vi "Client.vi"   [LabVIEW 2013]
uses:
  <vilib>/NXT/Block Support/NXT_MessageMailbox.ctl
  <vilib>/NXT/Dual Mode Library/Display/drawText.vi
  <vilib>/NXT/Dual Mode Library/BT/BlueTooth_Write_String.vi
types:
  T1 = typedef "LVHSConnector.ctl" = refnum<class "BrickReference.lvclass">
  T2 = typedef "NXT_MessageMailbox.ctl" = u8
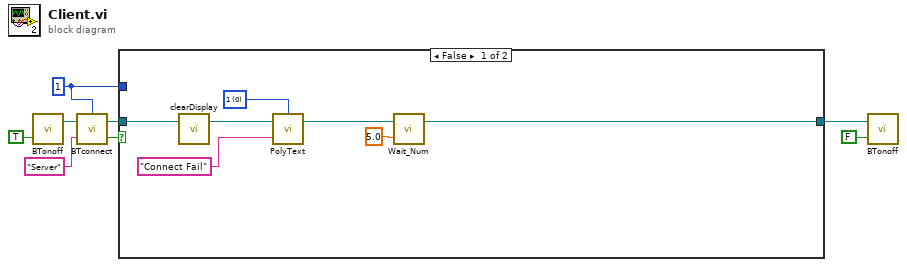
[diagram p0: block diagram]
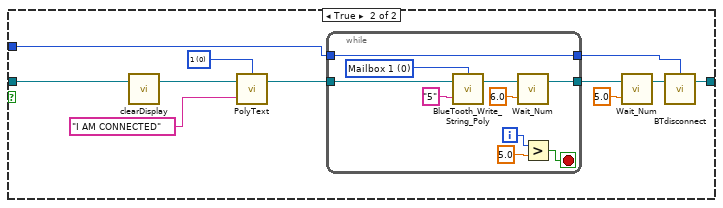
[diagram p2: hidden frame]
diagram:
  w5 = u8 1 ("Connection")
  n1 = call <vilib>:"BTonoff.vi"("On/Off"=TRUE) -> ("NXT/EV3"=w8:T1)  [unwired: 2 in, 1 out]
  n2 = call <vilib>:"BTconnect.vi"("Partner Name"="Server", "NXT/EV3"=w8, "Connection"=w5) -> ("Success"=w2:bool, "NXT/EV3"=w3:T1)
  n3 = case shown="False" w2 {
    tunnel: w5 -> [_ w19]
    tunnel: [w9 w26] -> w4
    tunnel: w3 -> [w10 w20]
    frame False {
      w13 = i16 0 items=["1", "2", "3", "4", "5", "6", "7", "8", "9", "10", "11", "12"] ("Line")
      n4 = call <vilib>:"clearDisplay.vi"("NXT/EV3"=w10) -> ("NXT/EV3"=w15:T1)  [unwired: 3 in]
      n5 = call-poly <vilib>:"PolyText.vi"("Text"="Connect Fail", "NXT/EV3"=w15, "Line"=w13) -> ("NXT/EV3"=w14:T1)  [unwired: 1 in]
      n6 = call <vilib>:"Wait_Num.vi"("Time (1 sec)"=sgl 5.0, "NXT/EV3"=w14) -> ("NXT/EV3"=w9:T1)  [unwired: 2 in]
    }
    frame True {
      w24 = i16 0 items=["1", "2", "3", "4", "5", "6", "7", "8", "9", "10", "11", "12"] ("Line")
      n7 = call <vilib>:"clearDisplay.vi"("NXT/EV3"=w20) -> ("NXT/EV3"=w25:T1)  [unwired: 3 in]
      n8 = call-poly <vilib>:"PolyText.vi"("Text"="I AM CONNECTED", "NXT/EV3"=w25, "Line"=w24) -> ("NXT/EV3"=w17:T1)  [unwired: 1 in]
      n9 = while {
        tunnel: w19 -> [w28]
        tunnel: [w30] -> w18
        tunnel: w17 -> [w35]
        tunnel: [w28] -> w16
        i -> [w33]
        stop <- w32 stop-if-true
        w27 = T2 0 items=["Mailbox 1", "Mailbox 2", "Mailbox 3", "Mailbox 4", "Mailbox 5", "Mailbox 6", "Mailbox 7", "Mailbox 8", "Mailbox 9", "Mailbox 10"] ("Mailbox")
        n10 = call-poly <vilib>:"BlueTooth_Write_String_Poly.vi"("Message"="5", "NXT/EV3"=w35, "Mailbox"=w27) -> ("NXT/EV3"=w31:T1)  [unwired: 1 in]
        n11 = call <vilib>:"Wait_Num.vi"("Time (1 sec)"=sgl 6.0, "NXT/EV3"=w31) -> ("NXT/EV3"=w30:T1)  [unwired: 2 in]
        n12 = Greater?(x=w33, y=5.0) -> (0:w32:bool)
      }
      n13 = call <vilib>:"Wait_Num.vi"("Time (1 sec)"=sgl 5.0, "NXT/EV3"=w18) -> ("NXT/EV3"=w21:T1)  [unwired: 2 in]
      n14 = call <vilib>:"BTdisconnect.vi"("NXT/EV3"=w21, "Connection"=w16) -> ("NXT/EV3"=w26:T1)  [unwired: 1 in, 1 out]
    }
  }
  n15 = call <vilib>:"BTonoff.vi"("On/Off"=FALSE, "NXT/EV3"=w4) -> ()  [unwired: 1 in, 2 out]
